vi "Wind Turbine Create.vi"(8 "error in (no error)":errorcluster, 11 "SEQ Name":string) -> (0 "error out":errorcluster, 3 "Data Refnum out":T1)   [LabVIEW 2009, in "SEQ - Solution.lvlib"]
doc: "One VI in the solution for the Wind Turbine class. This group of VIs is built on the SEQ design pattern and illustrates the power of references and named queues.\n\nAAL 9/09"
uses:
  SEQ - Solution.lvlib
  Controls/Wind Turbine Data.ctl
  Controls/Wind Turbine DataRef.ctl
panel:
  in  "default":T2
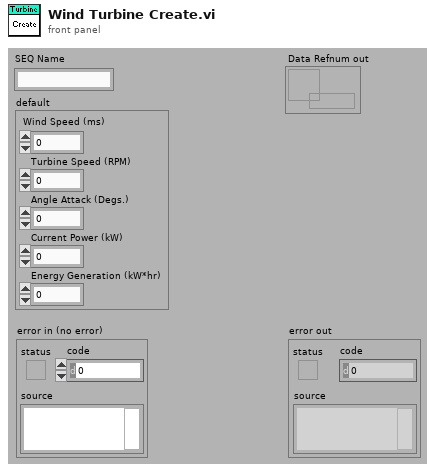
[diagram p1: front panel]
types:
  T1 = typedef "SEQ - Solution.lvlib/Wind Turbine DataRef.ctl" = refnum<queue>
  T2 = typedef "SEQ - Solution.lvlib/Wind Turbine Data.ctl" = cluster{" Wind Speed (ms)":dbl, "Turbine Speed (RPM)":dbl, "Angle Attack (Degs.)":dbl, "Current Power (kW)":dbl, "Energy Generation (kW*hr)":dbl}
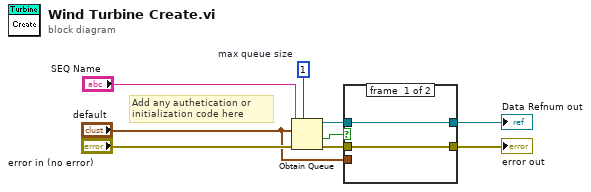
[diagram p0: block diagram]
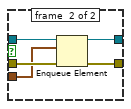
[diagram p2: hidden frame]
diagram:
  w8 = 1  # max queue size
  # "Add any authetication or\ninitialization code here"
  n1 = Obtain Queue(max queue size (-1, unlimited)=w8, name (unnamed)="SEQ Name", element data type="default", error in (no error)="error in (no error)") -> (queue out=w5:refnum<queue>, created new?=w1:bool, error out=w6:errorcluster)  [unwired: 1 in]
  n2 = case shown="False" w1 {
    tunnel: w6 -> [w10 w16]
    tunnel: w5 -> [w11 w15]
    tunnel: [w10 w14] -> w4
    tunnel: "default" -> [_ w13]
    tunnel: [w11 w12] -> w2
    frame #0 {
    }
    frame #1 {
      n3 = Enqueue Element(queue=w15, element=w13, error in (no error)=w16) -> (queue out=w12:refnum<queue>, error out=w14:errorcluster)  [unwired: 2 out]
    }
  }
  "error out" <- w4
  "Data Refnum out" <- w2
